vi "Hardware-DI-A Pump Ref Setup-Host.vi"() -> ()   [LabVIEW 2016]
panel:
  in  "RefPumpVoltageOffset":sgl
  in  "RefPumpVoltageMultiplier":sgl
  in  "RefPumpCurrentOffset":sgl
  in  "RefPumpCurrentMultiplier":sgl
  in  "RefPumpTimeAxisOffset":sgl
  in  "RefPumpTimeAxisMultiplier":sgl
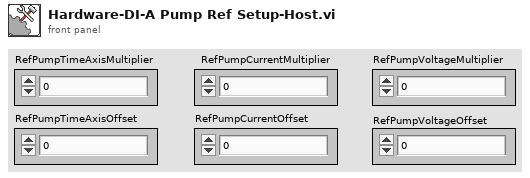
[diagram p1: front panel]
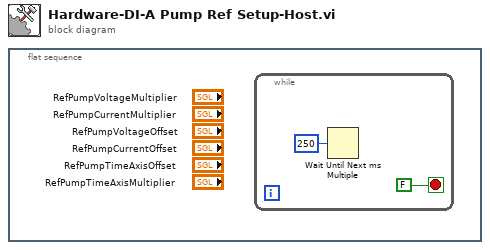
[diagram p0: block diagram]
diagram:
  n1 = flat-sequence {
    frame #0 {
      n2 = while {
        stop <- FALSE stop-if-true
        n3 = Wait Until Next ms Multiple(millisecond multiple=u32 250) -> ()  [unwired: 1 out]
      }
    }
  }
